vi "Create Test Configuration.vi"() -> (0 "error out":errorcluster, 1 "Names":string[](array[string]), 2 "error classifications":T1[](array[typedef])=[{"code"=-1, "error classification"=enum."unknown"}, {"code"=7, "error classification"=enum."critical"}, {"code"=1984, "error classification"=enum."recoverable"}], 3 "Module":refnum<class "user control module configuration.lvclass">, 4 "Channels":refnum<class "TBM channel.lvclass">[](array[class]), 5 "instance identifier":string)   [LabVIEW 2014, in "User Control Module Test.lvlib"]
uses:
  User Control Module Test.lvlib
  <vilib>/NI/Tag Bus Module Framework/channel/TBM channel.lvclass
  module/configuration/user control module configuration.lvclass
  <vilib>/NI/DCAF/Tag Editor Core/control module/configuration/error classification setting.ctl
  <vilib>/NI/Tag Bus Module Framework/runtime/error classification.ctl
  <vilib>/NI/Tag Bus/tag/tag descriptor.lvclass/tag descriptor.ctl
  <vilib>/NI/DCAF/Tag Editor Core/control module/configuration/control module configuration.lvclass/control module configuration.ctl
  <vilib>/NI/DCAF/Tag Editor Core/control module/configuration/Write configured channels.vi
  <vilib>/NI/DCAF/Tag Editor Core/control module/configuration/Write error classifications.vi
  <vilib>/NI/Configuration Framework/serializable configuration/NISE_CEF_serializable configuration.lvclass
  <vilib>/NI/DCAF/Tag Editor Core/control module/configuration/control module configuration.lvclass
  <vilib>/NI/Tag Bus/tag/tag descriptor.lvclass
  <vilib>/NI/Tag Bus Module Framework/runtime/TBM module execution interface.lvclass
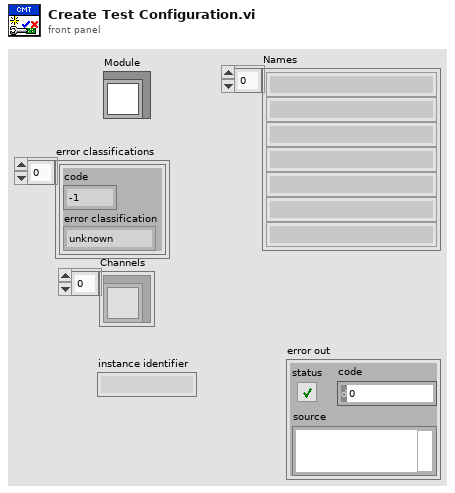
[diagram p1: front panel]
types:
  T1 = typedef "control module configuration.lvclass/error classification setting.ctl" = cluster{"code":i32, "error classification":T2}
  T2 = typedef "TBM module execution interface.lvclass/error classification.ctl" = enum16{"unknown", "none", "trivial", "recoverable", "critical"}
  T3 = cluster{"channel":refnum<class "TBM channel.lvclass">}
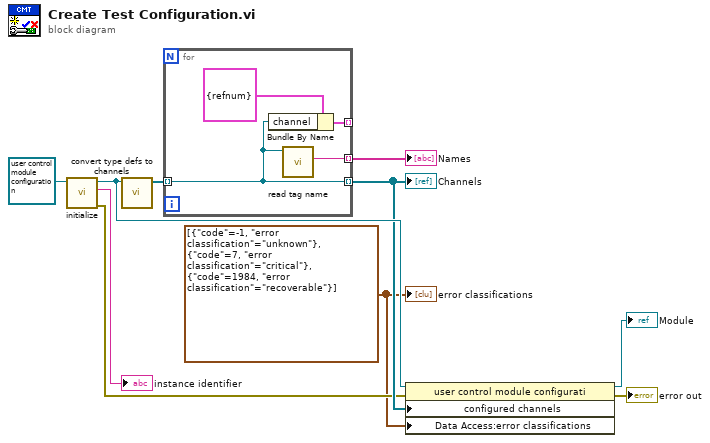
[diagram p0: block diagram]
diagram:
  w1 = T1[] [{"code"=-1, "error classification"=enum."unknown"}, {"code"=7, "error classification"=enum."critical"}, {"code"=1984, "error classification"=enum."recoverable"}] ("error classifications")
  n1 = call <vilib>:"initialize.vi"("configuration in"=refnum<class "user control module configuration.lvclass"> refnum ("user control module configuration")) -> ("error out"=w2:errorcluster, "identifier"=→"instance identifier":string, "configuration out"=w4:refnum<class "user control module configuration.lvclass">)  [unwired: 8 in]
  n2 = call <vilib>:"convert type defs to channels.vi"("fixed channel configuration"=w4) -> ("Array out"=w5:refnum<class "TBM channel.lvclass">[])  [unwired: 9 in, 1 out]
  n3 = for {
    tunnel: [w14] -> _ mode=indexing
    tunnel: [w11] -> w9 mode=indexing
    tunnel: [w12] -> w3 mode=indexing
    tunnel: w5 -> [w12] mode=indexing
    n4 = Bundle By Name(cluster=T3 {"channel"=refnum} ("Line"), "channel"=w12) -> (w14:T3)
    n5 = call <vilib>:"read tag name.vi"("system tag in"=w12) -> ("name"=w11:string)  [unwired: 8 in, 2 out]
  }
  "Names" <- w9
  "Channels" <- w3
  n6 = property class="user control module configurati"(reference=w4, error in=w2, "configured channels"=w3, "Data Access:error classifications"=w1) -> (reference out=→"Module":refnum<class "user control module configuration.lvclass">, error out=→"error out":errorcluster)
  "error classifications" <- w1
